vi "GFGreadAllFromFile.vi"(8 "error in":errorcluster, 11 "file path":path) -> (0 "error out":errorcluster)   [LabVIEW 2012, in "GFG library.lvlib"]
doc: "SciScan 1.2 160622"
uses:
  <vilib>/Utility/VariantDataType/Type.ctl
  GFG library.lvlib
  <vilib>/Utility/VariantDataType/VariantType.lvlib
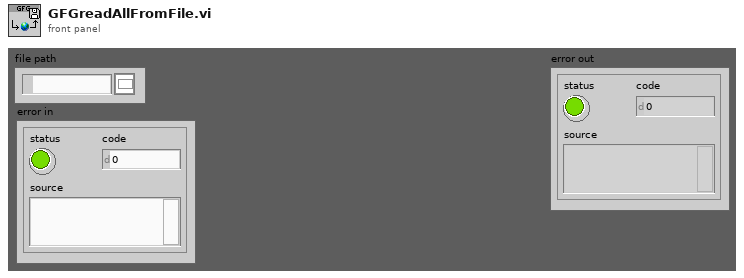
[diagram p1: front panel]
types:
  T1 = typedef "VariantType.lvlib/Type.ctl" = enum8{"Invalid Type", "Void", "I8", "I16", "I32", "I64", "U8", "U16", "U32", "U64", "Single Float", "Double Float", "Extended Float", "Single Complex", "Double Complex", "Extended Complex", "Enum U8", "Enum U16", "Enum U32", "Enum U64", "Single Float With Unit", "Double Float With Unit", "Extended Float With Unit", "Single Complex with Unit", "Double Complex with Unit", "Extended Complex with Unit", "Boolean", "String", "Path", "Picture", "Tag", "Array", "Cluster", "Variant", "LV Variant", "Waveform", "Timestamp", "Digital Waveform", "Digital Data", "ExpressData", "Refnum", "External Data", "VI", "Poly VI", "LabVIEW Class Instance", "Fixed Point"}
  T2 = cluster{"Variable Name Out":string, "Data Type Out":T1, "Variant Out":variant}[]
  T3 = enum16{"open", "replace", "create", "open or create", "replace or create", "replace or create with confirmation"}
  T4 = cluster{"Array of Clusters of Variables":cluster{"Variable Name Out":string, "Data Type Out":T1, "Variant Out":variant}[]}[]
  T5 = cluster{"Array of Clusters of Variables":cluster{"Variable Name Out":string, "Data Type Out":T1, "Variant Out":variant}[]}
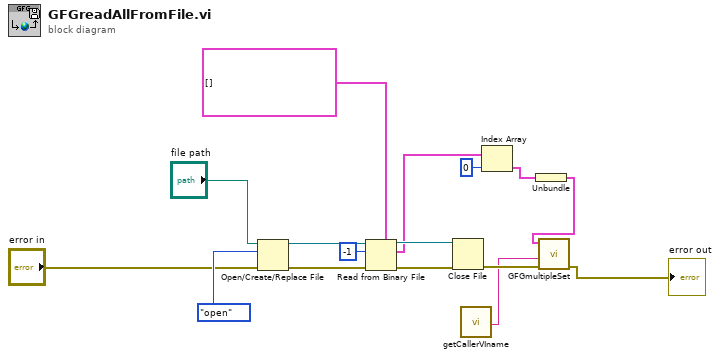
[diagram p0: block diagram]
diagram:
  n1 = Open/Create/Replace File(file path (use dialog)="file path", error in="error in", operation (0:open)=T3."open") -> (refnum out=w15:refnum<file>, error out=w13:errorcluster)  [unwired: 3 in, 1 out]
  n2 = Read from Binary File(5:T2 [] ("Array of Clusters of Variables"), 8:w13, 10:-1 ("count (1)"), 11:w15) -> (0:w12:errorcluster, 2:w5:T4, 3:w11:refnum<file>)  [unwired: 2 in, 1 out]
  n3 = Close File(refnum=w11, error in=w12) -> (error out=w7:errorcluster)  [unwired: 1 out]
  n4 = call "getCallerVIname.vi"() -> ("VI name"=w1:string)  [unwired: 19 in]
  n5 = Index Array(array=w5, index=0) -> (element=w3:T5)
  n6 = Unbundle(w3) -> ("Array of Clusters of Variables"=w2:T2)
  n7 = call "GFGmultipleSet.vi"("error in (no error)"=w7, "Source VI"=w1, "Array of Clusters of Variables"=w2) -> ("error out"=→"error out":errorcluster)  [unwired: 8 in]
